vi "generate transactions.vi"() -> ()   [LabVIEW 2019]
uses:
  <vilib>/numeric/Random Number (Range) U64.vi
  <vilib>/numeric/sub_Random U32.vi
panel:
  in  "Min number of items":u64=2
  in  "Max number of items":u64=10
  in  "Number of files":i32=5
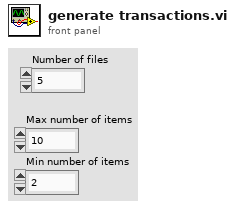
[diagram p1: front panel]
types:
  T1 = enum16{"open", "replace", "create", "open or create", "replace or create", "replace or create with confirmation"}
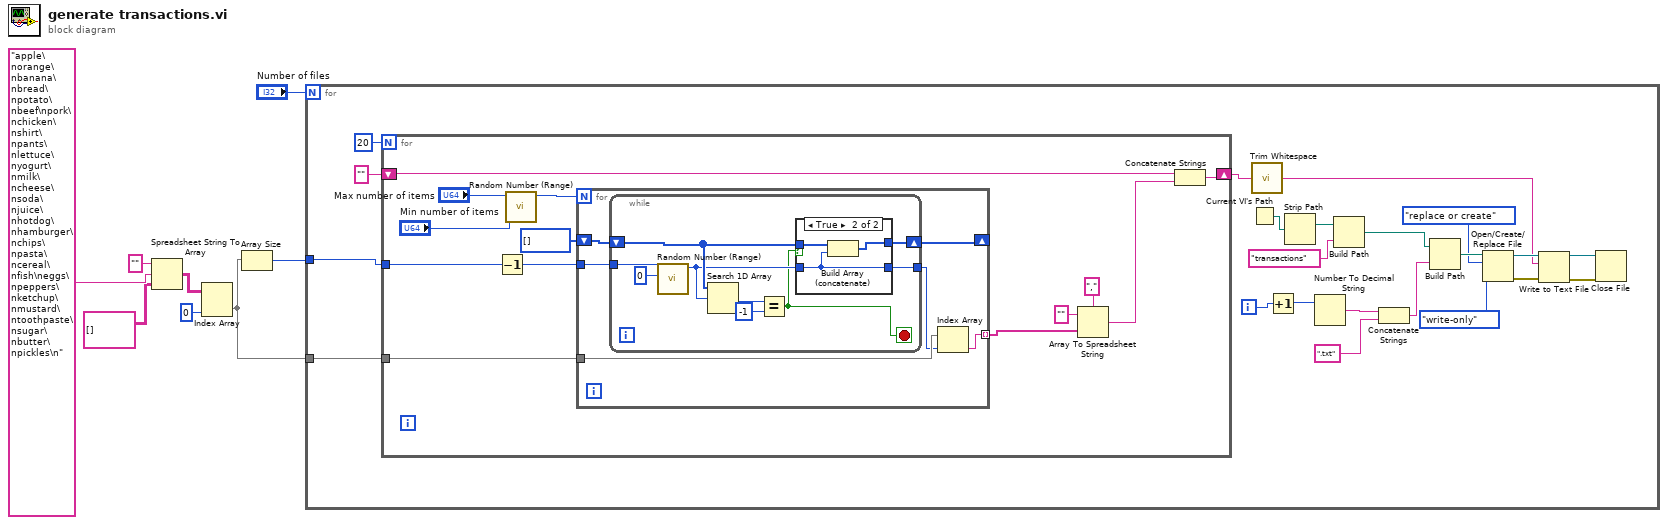
[diagram p0: block diagram]
diagram:
  n1 = Spreadsheet String To Array(format string="", spreadsheet string="apple\norange\nbanana\nbread\npotato\nbeef\npork\nchicken\nshirt\npants\nlettuce\nyogurt\nmilk\ncheese\nsoda\njuice\nhotdog\nhamburger\nchips\npasta\ncereal\nfish\neggs\npeppers\nketchup\nmustard\ntoothpaste\nsugar\nbutter\npickles\n", array type (2D Dbl)=string[][] []) -> (array=w5:string[][])  [unwired: 1 in]
  n2 = Index Array(array=w5, index (col)=0 ("disabled index (col)")) -> (element=w3:string[])  [unwired: 1 in]
  n3 = Array Size(array=w3) -> (size(s)=w2:i32)
  n4 = for {
    N: "Number of files" -> [_]
    tunnel: w3 -> [w30]
    tunnel: w2 -> [w28]
    i -> [w21]
    n5 = for {
      N: 20 -> [_]
      tunnel: w30 -> [w42]
      tunnel: w28 -> [w39]
      shift-right: [w35] -> w26
      shift-left: "" -> [w34]
      n6 = Decrement(x=w39) -> (x-1=w41:i32)
      n7 = call-poly <vilib>:"Random Number (Range).vi"("lower bound (0)"="Min number of items", "upper bound (100)"="Max number of items") -> ("number"=w43:u64)  [unwired: 9 in]
      n8 = for {
        N: w43 -> [_]
        tunnel: w41 -> [w49]
        tunnel: w42 -> [w46]
        tunnel: [w44] -> w32 mode=indexing
        shift-right: [w47] -> _
        shift-left: u64[] [] ("number") -> [w48]
        n9 = while {
          tunnel: w49 -> [w58]
          shift-right: [w56] -> w47
          shift-left: w48 -> [w55]
          tunnel: [w50] -> w45
          stop <- w51 stop-if-true
          n10 = call-poly <vilib>:"Random Number (Range).vi"("lower bound (0)"=u64 0 ("lower bound (-100)"), "upper bound (100)"=w58) -> ("number"=w54:u64)  [unwired: 9 in]
          n11 = Search 1D Array(1D array=w55, element=w54) -> (index of element=w53:i32)  [unwired: 1 in]
          n12 = Equal?(x=w53, y=-1) -> (x = y?=w51:bool)
          n13 = case shown="True" w51 {
            tunnel: w55 -> [w60 w63]
            tunnel: w54 -> [w59 w61]
            tunnel: [w60 w62] -> w56
            tunnel: [w59 w61] -> w50
            frame False {
            }
            frame True {
              n14 = Build Array (concatenate)(w63, w61) -> (w62:u64[])
            }
          }
        }
        n15 = Index Array(array=w46, index=w45) -> (element=w44:string)
      }
      n16 = Array To Spreadsheet String(delimiter (Tab)=",", array=w32, 3:"" ("format string")) -> (spreadsheet string=w33:string)
      n17 = Concatenate Strings(w34, w33) -> (w35:string)
    }
    n18 = Current VI's Path() -> (path=w25:path)
    n19 = call <vilib>:"Trim Whitespace.vi"("string"=w26) -> ("trimmed string"=w11:string)  [unwired: 1 in]
    n20 = Increment(x=w21) -> (x+1=w20:i32)
    n21 = Strip Path(path=w25) -> (stripped path=w24:path)  [unwired: 1 out]
    n22 = Number To Decimal String(number=w20) -> (decimal integer string=w19:string)  [unwired: 1 in]
    n23 = Build Path(base path=w24, name or relative path="transactions") -> (appended path=w22:path)
    n24 = Concatenate Strings(w19, ".txt" ("string")) -> (w17:string)
    n25 = Build Path(base path=w22, name or relative path=w17) -> (appended path=w16:path)
    n26 = Open/Create/Replace File(file path (use dialog)=w16, operation (0:open)=T1."replace or create", access (0:read/write)=enum16{"read/write", "read-only", "write-only"}."write-only") -> (refnum out=w12:refnum<file>, error out=w13:errorcluster)  [unwired: 3 in, 1 out]
    n27 = Write to Text File(file (use dialog)=w12, text=w11, error in=w13) -> (refnum out=w9:refnum<file>, error out=w10:errorcluster)  [unwired: 1 in, 1 out]
    n28 = Close File(refnum=w9, error in=w10) -> ()  [unwired: 2 out]
  }
